vi "Statnett PMU Recorder Light.vi"(8 "error in (no error)":errorcluster) -> (0 "error out":errorcluster)   [LabVIEW 2013, in "PMU Recorder Light.lvlib"]
uses:
  PMU Recorder Light.lvlib
  <vilib>/Platform/TimedLoop/XDataNode/timing_clust.ctl
  <vilib>/Platform/TimedLoop/XDataNode/nitl_modes.ctl
  <vilib>/Platform/TimedLoop/XDataNode/wakeup.ctl
  <vilib>/Utility/sysdir.llb/System Directory Type.ctl
  <vilib>/platform/TimedLoop/XDataNode/XDataNode.xnode
  Phasor Data Concentrator Class/Phasor Data Concentrator.lvclass
  <vilib>/Platform/TimedLoop/XDataNode/XDNodeRunTimeDep.lvlib
panel:
  out "Number of bad dt":u64
  out "Latest Time Stamp":timestamp format="%<%X  %x>T"
  in  "Channel Selector":bool
  out "Manual Control":bool
  out "PDC Initialized":bool
  out "Queue Active":bool
  out "Connected":bool
  out "Configuration File Read":bool
  out "PDC Connected":bool
  out "Shutdown":bool
  out "Autostart":bool
  out "Bad Data Removal":bool
  out "Buffer Active":bool
  out "Configuration File Timeout":bool
  out "Configuration File Received":bool
  out "Initializing...":bool
  out "Bad Data?":bool
  out "Complex Bad":dbl(knob) scale=0.0..50.0
  out "Writing To File Buffer?":bool
  out "Lost File Buffer Data?":bool
  out "Writer Activity":dbl(knob) scale=0.0..100.0
  out "Buffer Queued?":bool
  out "Reader Activity":dbl(knob) scale=0.0..100.0
  out "Data?":bool
  out "Bad dt?":bool
  in  "Raw Data Panel":bool
  out "Worker Status":bool
  out "Secretary Pulse":bool
  out "Quitting...":bool
  out "Status":string="off"
  out "Data Rate":sgl=nan format="%#_6f"
  out "Control":enum32{"Auto", "Manual"}(tab)
  in  "Config":bool
  in  "Restart":bool
  in  "Quit":bool
  in  "Shutdown Logging":bool
  in  "Pause":bool
  in  "Startup":bool
  in  "Abort Wait":bool
  in  "PDC Initialize":bool
  in  "DLL Start Readers":bool
  in  "DLL Shutdown":bool
  in  "DLL Read Config":bool
  in  "DLL Wait for config":bool
  in  "DLL Initialize":bool
  in  "Quit 2":bool
  in  "Restart 2":bool
  in  "Config 2":bool
  in  "dt min":dbl=nan
  in  "dt max":dbl=nan
  in  "PRL Configuration":T1={"Connection Settings"={"IP-address"="127.0.0.1", "Port"="5001", "ID Code"=1001}, "Autostart"=FALSE, "Bad Data Removal"=TRUE, "Access Buffer Active"=TRUE, "Wait for Config Total Time [ms]"=2000, "Seconds to Wait if Config Fails [s]"=10, "Live Data Buffer Size"=5, "Number of Live Buffers in Access Buffer"=0, "Data Rate History"=100, "Complex Data Points Allowed Equal"=10, "Analog Data Points Allowed Equal"=50, "Number of Connection Attempts"=0, "Access Queue Active"=FALSE, "Access Buffer Size [hh:mm]"=600.0, "Sampling rate [Hz]"=nan, "Manual Control"=FALSE, "dt Tolerance [microseconds]"=10.0, "Wait for Config Timeout [ms]"=20, "Max Time Stamp Age Before Reconnect [s]"=10.0, "Poll New Data Timeout [ms]"=5} {"Access Buffer Size [hh:mm]" format="%<%H:%M>t"}
  # "INPUT"
  # "OUTPUT"
  # "INTERMEDIATE"
  # "v1.2  2013-08-01"
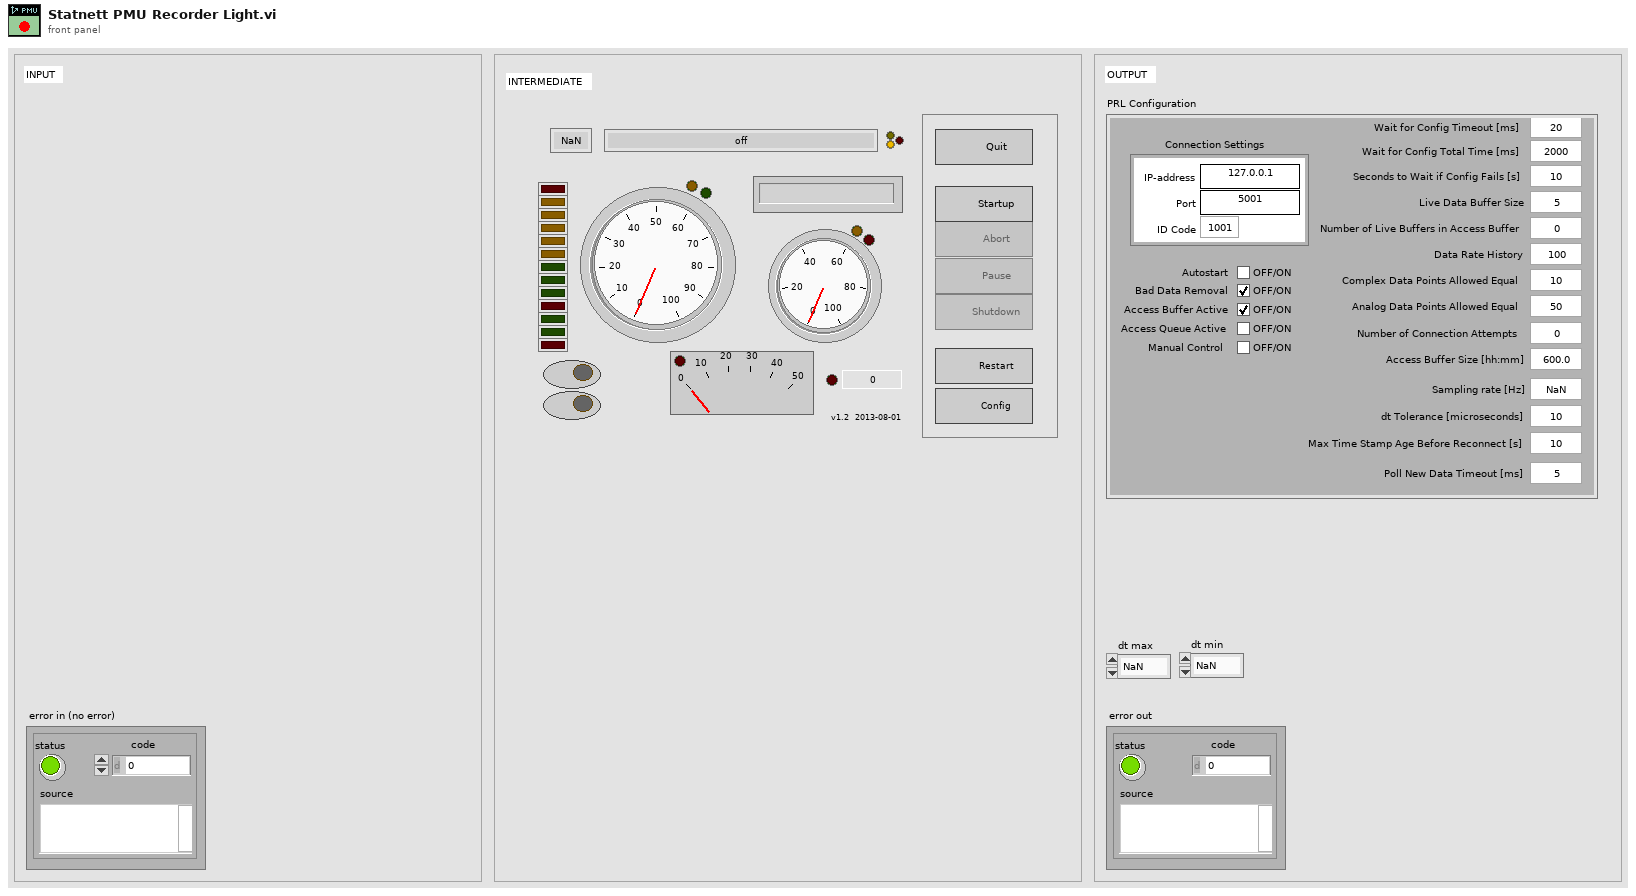
[diagram p1: front panel]
types:
  T1 = cluster{"Connection Settings":cluster{"IP-address":string, "Port":string, "ID Code":u32}, "Autostart":bool, "Bad Data Removal":bool, "Access Buffer Active":bool, "Wait for Config Total Time [ms]":i32, "Seconds to Wait if Config Fails [s]":i32, "Live Data Buffer Size":i32, "Number of Live Buffers in Access Buffer":i32, "Data Rate History":i32, "Complex Data Points Allowed Equal":i32, "Analog Data Points Allowed Equal":i32, "Number of Connection Attempts":i32, "Access Queue Active":bool, "Access Buffer Size [hh:mm]":dbl, "Sampling rate [Hz]":dbl, "Manual Control":bool, "dt Tolerance [microseconds]":dbl, "Wait for Config Timeout [ms]":i32, "Max Time Stamp Age Before Reconnect [s]":dbl, "Poll New Data Timeout [ms]":u16}
  T2 = typedef "XDNodeRunTimeDep.lvlib/timing_clust.ctl" = cluster{"Expected End [f-1]":u64, "Actual End [f-1]":u64, "Finished Late? [f-1]":bool, "Expected End [i-1]":u64, "Actual End [i-1]":u64, "Finished Late? [i-1]":bool, "Expected Start [i]":u64, "Actual Start [i]":u64, "Expected Start [f]":u64, "Actual Start [f]":u64, "Source Name":string, "Structure Name":string, "Period":i64, "Deadline":i64, "Offset":i64, "Start":i64, "Priority":i32, "Timeout":i32, "Mode":T3, "Wakeup Reason":T4, "Error":errorcluster, "Source Type":string, "Secondary Source Type":string, "Global End Time":u64, "Global Start Time":u64, "Frame Duration":u64, "Iteration Duration":u64, "Assigned CPU":i32, "I/O Scan Engine Mode":u32}
  T3 = typedef "XDNodeRunTimeDep.lvlib/nitl_modes.ctl" = enum32{"No Change", "Process missed periods, maintain original phase", "Discard missed periods, maintain original phase", "Process missed periods, ignore original phase", "Discard missed periods, ignore original phase"}
  T4 = typedef "XDNodeRunTimeDep.lvlib/wakeup.ctl" = enum32{"Normal", "Aborted", "Asynchronous wakeup", "Timing source error", "Timed loop error", "Timeout"}
  T5 = enum8{"Enabled", "Disabled", "Disabled and Grayed Out"}
  T6 = typedef "System Directory Type.ctl" = i32
  T7 = cluster{"IP-address":string, "Port":string, "ID Code":u32}
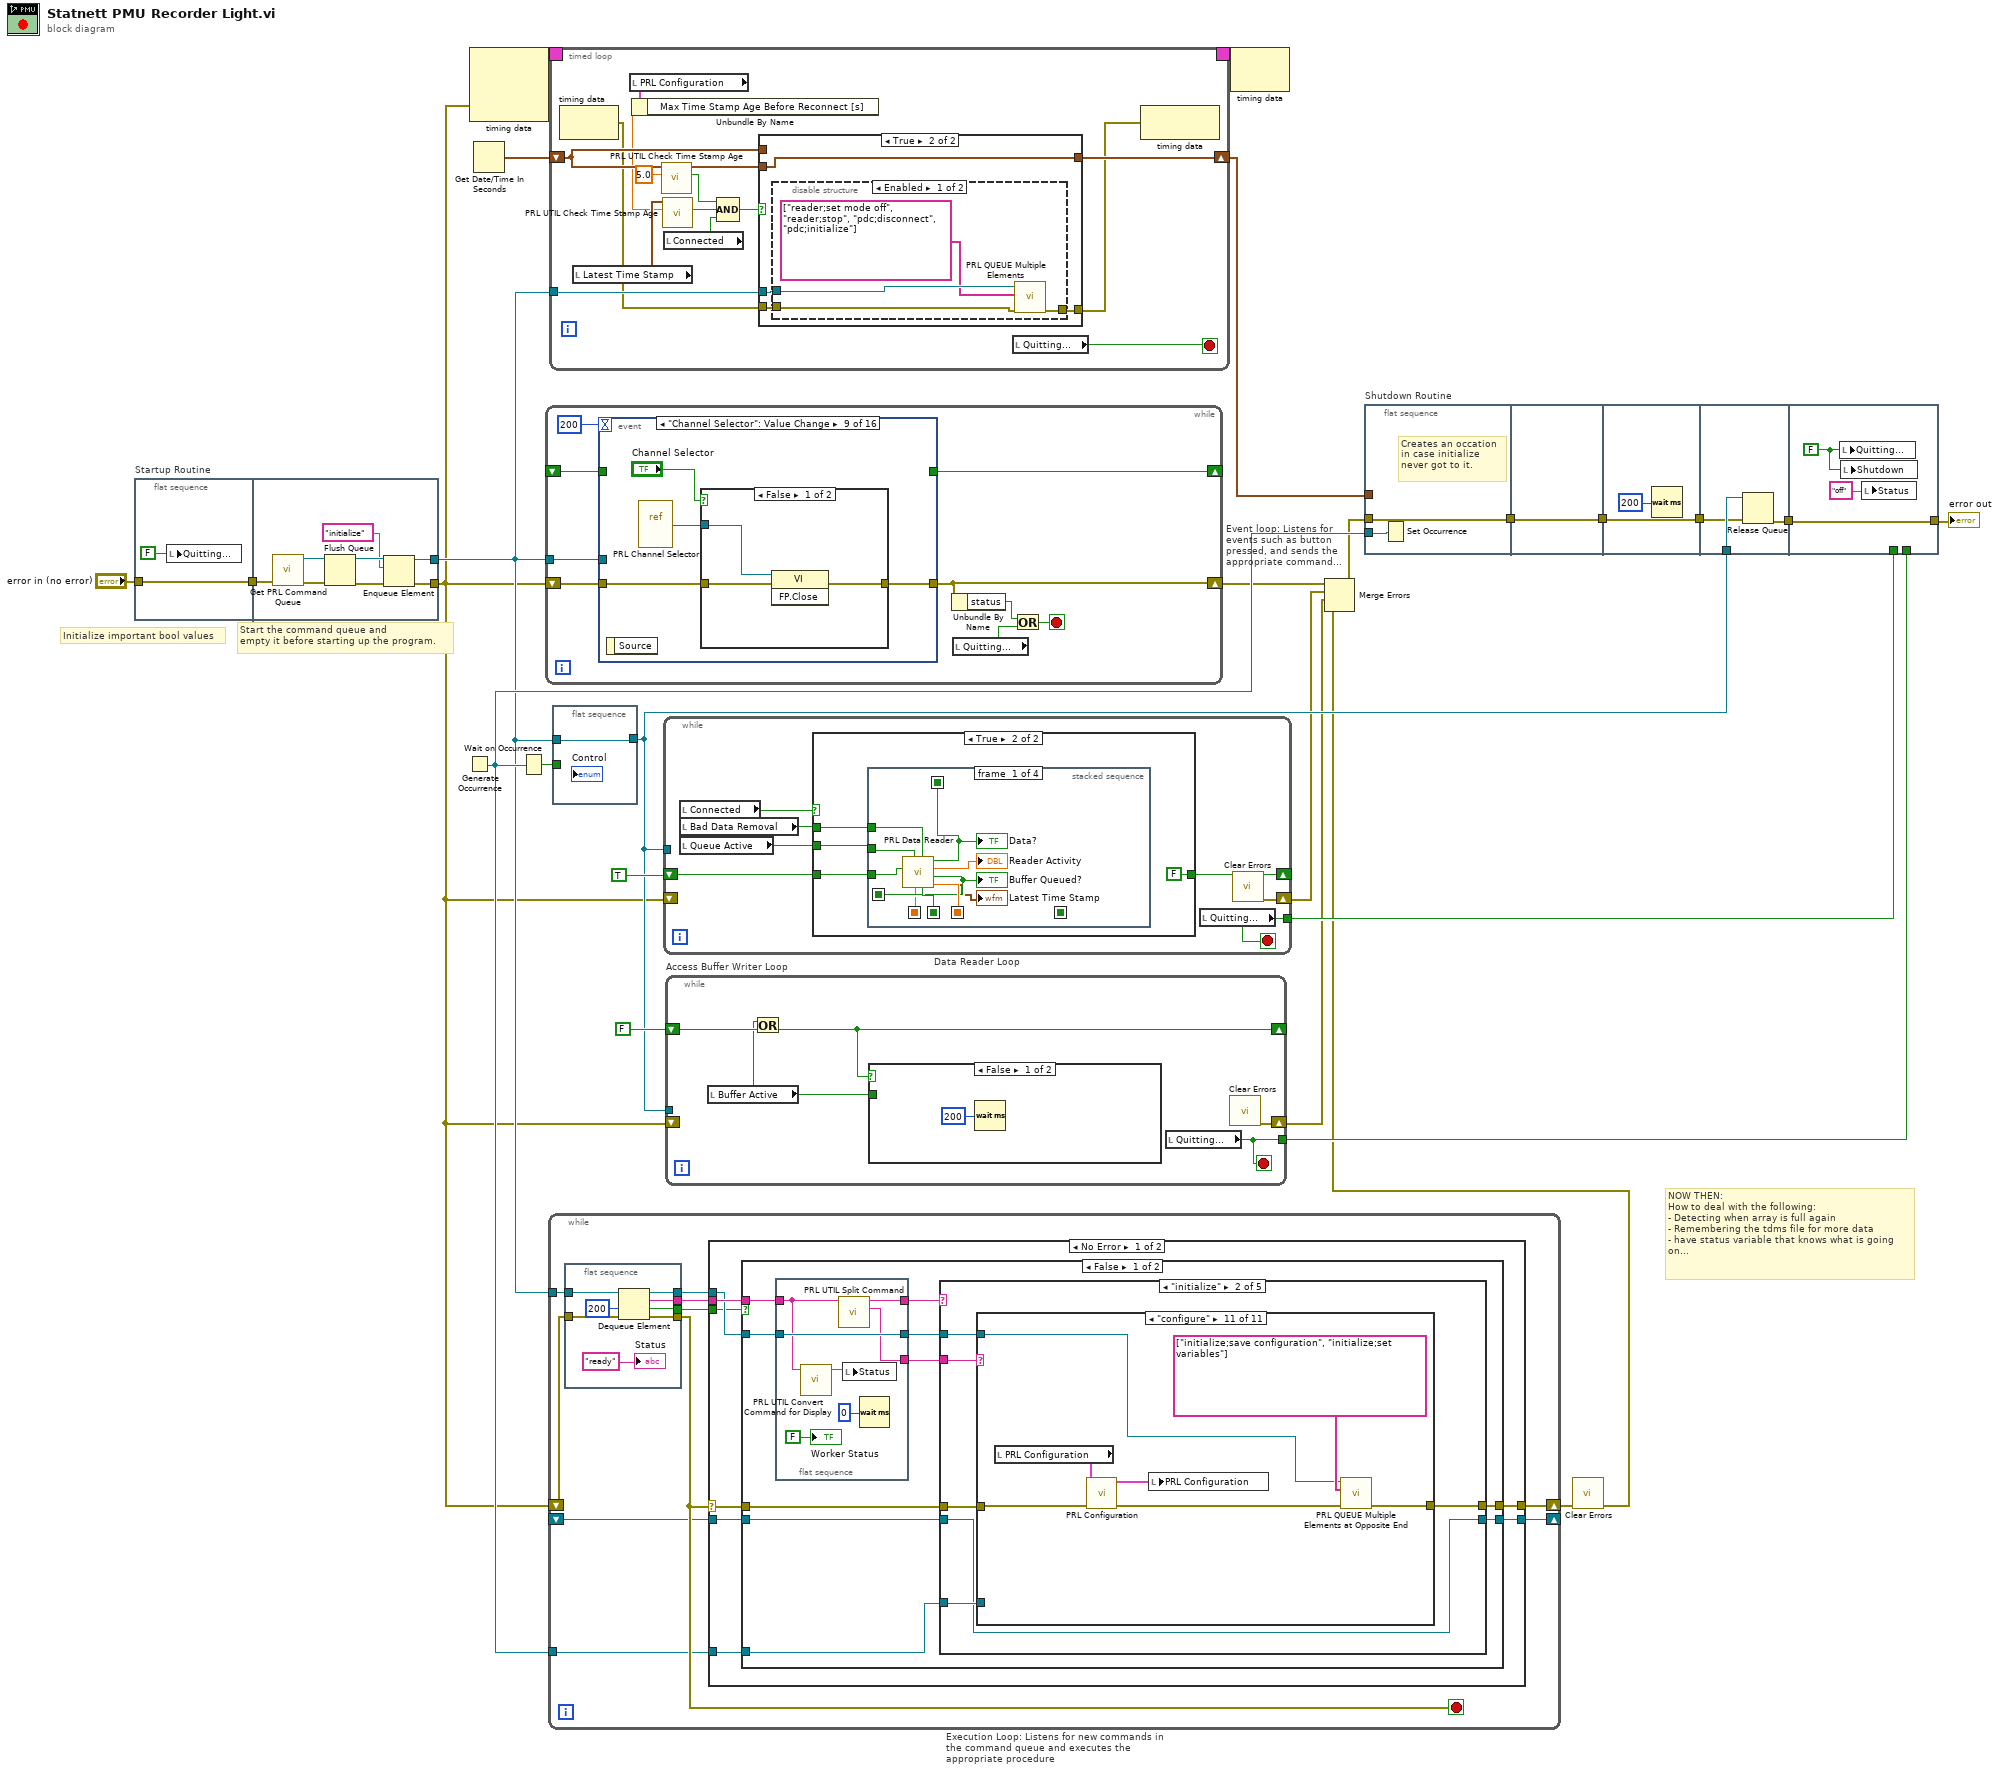
[diagram p0: block diagram]
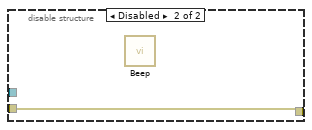
[diagram p3: hidden frame]
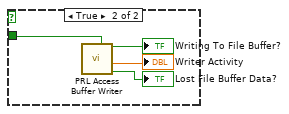
[diagram p4: hidden frame]
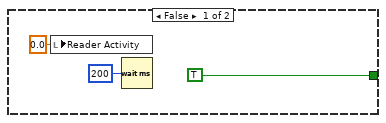
[diagram p5: hidden frame]
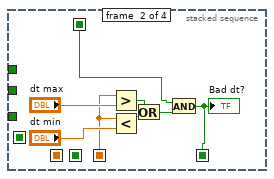
[diagram p6: hidden frame]
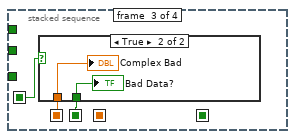
[diagram p7: hidden frame]
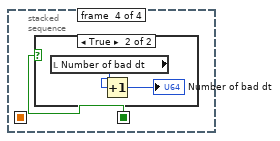
[diagram p9: hidden frame]
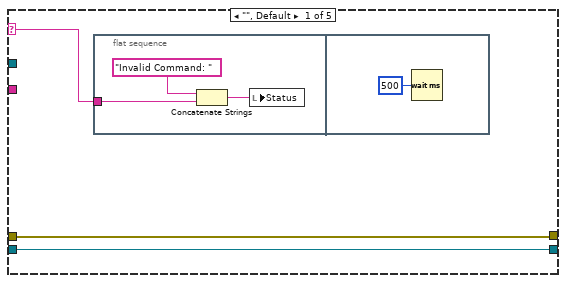
[diagram p11: hidden frame]
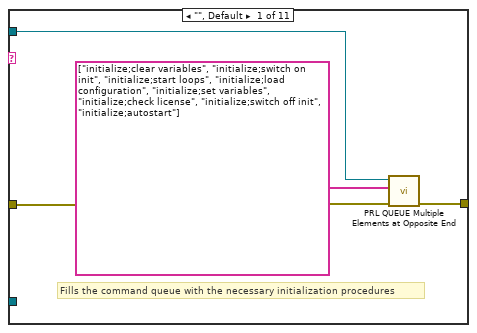
[diagram p12: hidden frame]
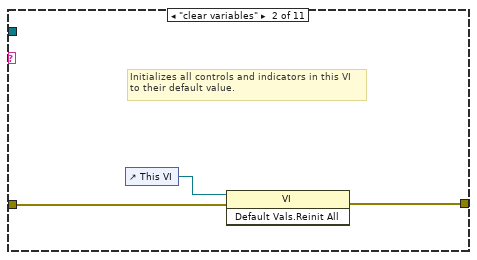
[diagram p13: hidden frame]
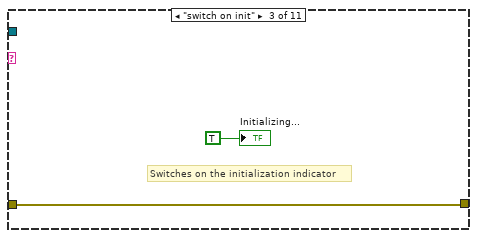
[diagram p14: hidden frame]
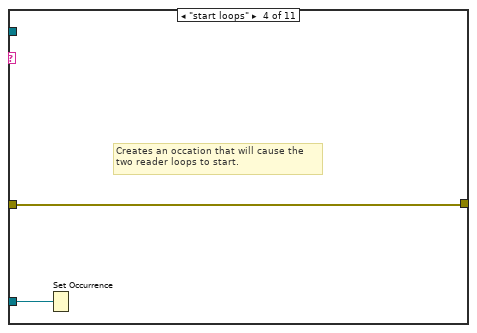
[diagram p15: hidden frame]
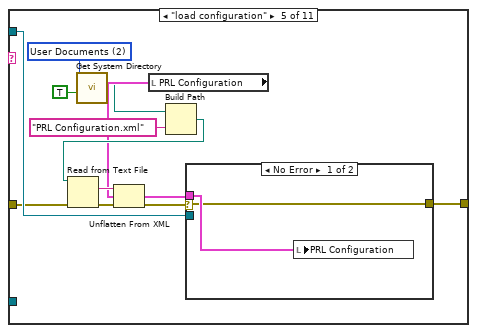
[diagram p16: hidden frame]
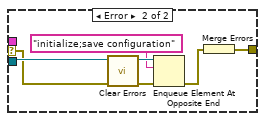
[diagram p17: hidden frame]
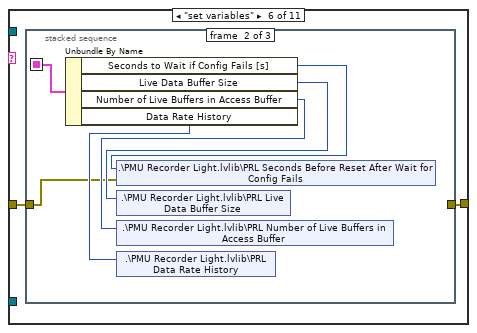
[diagram p18: hidden frame]
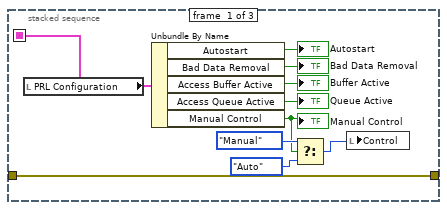
[diagram p19: hidden frame]
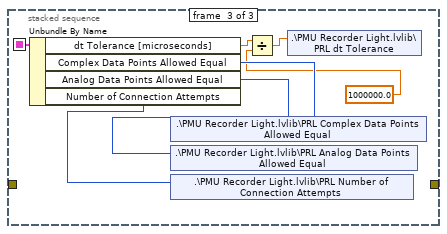
[diagram p20: hidden frame]
diagram:
  # "Initialize important bool values"
  # "Start the command queue and \nempty it before starting up the program."
  # "NOW THEN:\nHow to deal with the following:\n- Detecting when array is full again\n- Remembering the tdms file for more data\n- have status variable that knows what is going\non..."
  n1 = flat-sequence "Startup Routine" {
    tunnel: [w27] -> w14
    tunnel: "error in (no error)" -> [w27]
    tunnel: [w34] -> w10
    tunnel: [w32] -> w17
    tunnel: w14 -> [w29]
    frame #0 {
      n2 = local write "Quitting..."(FALSE ("Exit?")) -> ()
    }
    frame #1 {
      n3 = call "Get PRL Command Queue.vi"("error in (no error)"=w29) -> ("error out"=w30:errorcluster, "PRL Command Queue"=w31:refnum<queue>)  [unwired: 9 in]
      n4 = Flush Queue(queue=w31, error in (no error)=w30) -> (queue out=w35:refnum<queue>, error out=w36:errorcluster)  [unwired: 1 out]
      n5 = Enqueue Element(queue=w35, element="initialize", error in (no error)=w36) -> (queue out=w32:refnum<queue>, error out=w34:errorcluster)  [unwired: 2 out]
    }
  }
  n6 = Generate Occurrence() -> (w23:refnum<k4>)
  n7 = node-c288(w10) -> (w19:T2)  [unwired: 2 in]
  n8 = Get Date/Time In Seconds() -> (seconds since 1Jan1904=w16:timestamp)
  n9 = Wait on Occurrence(2:w23) -> (0:w24:bool)  [unwired: 2 in]
  n10 = while "Event loop: Listens for events such as button pressed, and sends the appropriate commands to the\ncommand queue" {
    shift-right: [w40] -> w9
    shift-left: w10 -> [w41]
    tunnel: w17 -> [w42]
    shift-right: [w37] -> _
    shift-left: _ -> [w38]
    stop <- w44 stop-if-true
    n11 = event shown="[8] \"Channel Selector\": Value Change" {
      selector: _ -> [_ _ _ _ _ _ _ _ _ _ _ _ _ _ _ _]
      dyn-events: _ -> [_ _ _ _ _ _ _ _ _ _ _ _ _ _ _ _]
      timeout: 200 -> [_ _ _ _ _ _ _ _ _ _ _ _ _ _ _ _]
      tunnel: w42 -> [_ w53 w57 w61 w65 w69 w76 _ _ w102 w106 w110 w114 w118 w122 w126]
      tunnel: [w48 w51 w55 w58 w63 w66 w74 w77 w88 w100 w103 w107 w112 w115 w119 w124] -> w40
      tunnel: w41 -> [w48 w52 w56 w59 w64 w67 w75 w78 w89 w101 w104 w108 w113 w116 w120 w125]
      tunnel: w38 -> [w47 _ _ _ _ _ _ _ _ _ _ _ _ _ _ _]
      tunnel: [w46 _ _ _ _ _ _ _ _ _ _ _ _ _ _ _] -> w37
      event Timeout {
        n12 = event-data() -> ()  [unwired: 3 out]
        n13 = Not(x=w47) -> (.not. x?=w46:bool)
        "Secretary Pulse" <- w47
      }
      event "Quit", "Quit 2": Value Change {
        n14 = event-data() -> ()  [unwired: 2 out]
        n15 = Enqueue Element(queue=w53, element="shutdown", error in (no error)=w52) -> (error out=w51:errorcluster)  [unwired: 3 out]
        "Shutdown" <- TRUE ("Shutdown")
      }
      event "Restart", "Restart 2": Value Change {
        n16 = event-data() -> ()  [unwired: 2 out]
        n17 = Enqueue Element(queue=w57, element="initialize", error in (no error)=w56) -> (error out=w55:errorcluster)  [unwired: 3 out]
      }
      event "Startup": Value Change {
        n18 = event-data() -> ()  [unwired: 2 out]
        n19 = call "PRL QUEUE Multiple Elements.vi"("error in"=w59, "Elements to Add"=string[] ["pdc;initialize"], "queue"=w61) -> ("error out"=w58:errorcluster)  [unwired: 7 in, 1 out]
      }
      event "PDC Initialize": Value Change {
        n20 = event-data() -> ()  [unwired: 2 out]
        n21 = Enqueue Element(queue=w65, element="pdc;init", error in (no error)=w64) -> (error out=w63:errorcluster)  [unwired: 3 out]
      }
      event "Shutdown Logging": Value Change {
        n22 = event-data() -> ()  [unwired: 2 out]
        n23 = call "PRL QUEUE Multiple Elements.vi"("error in"=w67, "Elements to Add"=string[] ["reader;set mode off", "reader;stop", "pdc;disconnect"], "queue"=w69) -> ("error out"=w66:errorcluster)  [unwired: 7 in, 1 out]
      }
      event "Pause": Value Change {
        n24 = event-data() -> ()  [unwired: 2 out]
        n25 = Select(t=string[] ["reader;set mode paused", "reader;stop"] ("Elements to Add"), s="Pause", f=string[] ["reader;start", "reader;set mode logging"] ("Elements to Add")) -> (s? t:f=w71:string[])
        n26 = call "PRL QUEUE Multiple Elements.vi"("error in"=w75, "Elements to Add"=w71, "queue"=w76) -> ("error out"=w74:errorcluster)  [unwired: 7 in, 1 out]
      }
      event "Raw Data Panel": Value Change {
        n27 = event-data() -> ()  [unwired: 2 out]
        n28 = vi-ref "PRL Raw Data Viewer.vi"() -> (w80:refnum<vi>)
        n29 = case shown="True" "Raw Data Panel" {
          tunnel: w80 -> [w83 w87]
          tunnel: [w82 w85] -> w77
          tunnel: w78 -> [w81 w84]
          frame False {
            n30 = invoke class="VI" method="FP.Close"(reference=w83, error in=w81) -> (error out=w82:errorcluster)  [unwired: 1 in, 2 out]
          }
          frame True {
            n31 = invoke class="VI" method="FP.Open"(reference=w87, error in=w84, "Activate"=TRUE ("Activate?")) -> (error out=w85:errorcluster)  [unwired: 2 in, 4 out]
          }
        }
      }
      event "Channel Selector": Value Change {
        n32 = event-data() -> ()  [unwired: 2 out]
        n33 = vi-ref "PRL Channel Selector.vi"() -> (w91:refnum<vi>)
        n34 = case shown="False" "Channel Selector" {
          tunnel: w91 -> [w94 w98]
          tunnel: [w93 w96] -> w88
          tunnel: w89 -> [w92 w95]
          frame False {
            n35 = invoke class="VI" method="FP.Close"(reference=w94, error in=w92) -> (error out=w93:errorcluster)  [unwired: 1 in, 2 out]
          }
          frame True {
            n36 = invoke class="VI" method="FP.Open"(reference=w98, error in=w95, "Activate"=TRUE ("Activate?")) -> (error out=w96:errorcluster)  [unwired: 2 in, 4 out]
          }
        }
      }
      event "Config", "Config 2": Value Change {
        n37 = event-data() -> ()  [unwired: 2 out]
        n38 = Enqueue Element(queue=w102, element="initialize;configure", error in (no error)=w101) -> (error out=w100:errorcluster)  [unwired: 3 out]
      }
      event "DLL Initialize": Value Change {
        n39 = event-data() -> ()  [unwired: 2 out]
        n40 = Enqueue Element(queue=w106, element="pdc;dll initialize", error in (no error)=w104) -> (error out=w103:errorcluster)  [unwired: 3 out]
      }
      event "DLL Wait for config": Value Change {
        n41 = event-data() -> ()  [unwired: 2 out]
        n42 = Enqueue Element(queue=w110, element="pdc;dll wait for config", error in (no error)=w108) -> (error out=w107:errorcluster)  [unwired: 3 out]
      }
      event "DLL Start Readers": Value Change {
        n43 = event-data() -> ()  [unwired: 2 out]
        n44 = Enqueue Element(queue=w114, element="pdc;start data readers", error in (no error)=w113) -> (error out=w112:errorcluster)  [unwired: 3 out]
      }
      event "DLL Read Config": Value Change {
        n45 = event-data() -> ()  [unwired: 2 out]
        n46 = Enqueue Element(queue=w118, element="pdc;dll read config", error in (no error)=w116) -> (error out=w115:errorcluster)  [unwired: 3 out]
      }
      event "DLL Shutdown": Value Change {
        n47 = event-data() -> ()  [unwired: 2 out]
        n48 = Enqueue Element(queue=w122, element="pdc;disconnect", error in (no error)=w120) -> (error out=w119:errorcluster)  [unwired: 3 out]
      }
      event "Abort Wait": Value Change {
        n49 = event-data() -> ()  [unwired: 2 out]
        n50 = Enqueue Element(queue=w126, element="reader;set mode startup", error in (no error)=w125) -> (error out=w124:errorcluster)  [unwired: 3 out]
      }
    }
    n51 = Unbundle By Name(w40) -> ("status"=w45:bool)
    n52 = local read "Quitting..."() -> (w43:bool)
    n53 = Or(x=w45, y=w43) -> (x .or. y?=w44:bool)
  }
  n54 = while "Execution Loop: Listens for new commands in the command queue and executes the appropriate procedure" {
    tunnel: w17 -> [w136]
    tunnel: w23 -> [w131]
    shift-right: [w129] -> _
    shift-left: _ -> [w130]
    shift-right: [w127] -> w2
    shift-left: w10 -> [w128]
    stop <- w133 stop-if-true
    n55 = flat-sequence {
      tunnel: w136 -> [w144]
      tunnel: [w143] -> w135
      tunnel: [w142] -> w134
      tunnel: [w141] -> w133
      tunnel: [w138] -> w132
      tunnel: w128 -> [w137]
      frame #0 {
        n56 = Dequeue Element(queue=w144, timeout in ms (-1)=200, error in (no error)=w137) -> (queue out=w143:refnum<queue>, element=w142:string, timed out?=w138:bool, error out=w141:errorcluster)
        "Status" <- "ready" ("Status")
      }
    }
    n57 = case shown="No Error" w133 {
      selector: w133 -> [w146 w502]
      tunnel: w135 -> [w151 _]
      tunnel: w134 -> [w152 _]
      tunnel: w132 -> [w150 _]
      tunnel: w131 -> [w149 _]
      tunnel: w130 -> [w148 w503]
      tunnel: [w147 w503] -> w129
      tunnel: [w145 w502] -> w127
      frame No Error {
        n58 = case shown="False" w150 {
          tunnel: w152 -> [w162 _]
          tunnel: w151 -> [w161 _]
          tunnel: w149 -> [w157 _]
          tunnel: w148 -> [w156 w499]
          tunnel: [w155 w499] -> w147
          tunnel: w146 -> [w154 w498]
          tunnel: [w153 w498] -> w145
          frame False {
            n59 = flat-sequence {
              tunnel: [w495] -> w160
              tunnel: w162 -> [w493]
              tunnel: w161 -> [w497]
              tunnel: [w497] -> w159
              tunnel: [w494] -> w158
              frame #0 {
                n60 = call "PRL UTIL Convert Command for Display.vi"("Command In"=w493) -> ("Command Out"=w492:string)  [unwired: 10 in]
                n61 = call "PRL UTIL Split Command.vi"("Command"=w493) -> ("Parameters"=w494:string, "Command Out"=w495:string)  [unwired: 9 in]
                n62 = local write "Status"(w492) -> ()
                n63 = Wait (ms)(milliseconds to wait=u32 0) -> ()  [unwired: 1 out]
                "Worker Status" <- FALSE ("System Ready")
              }
            }
            n64 = case shown="\"initialize\"" w160 {
              selector: w160 -> [w165 _ _ _ _]
              tunnel: w159 -> [_ w175 w269 w421 w482]
              tunnel: w158 -> [_ w174 w270 w422 w481]
              tunnel: w157 -> [_ w173 _ _ _]
              tunnel: w156 -> [w164 w172 w268 w420 w480]
              tunnel: [w164 w172 w267 w420 w480] -> w155
              tunnel: w154 -> [w163 w171 w266 w419 w479]
              tunnel: [w163 w170 w265 w418 w478] -> w153
              frame "", Default {
                n65 = flat-sequence {
                  tunnel: w165 -> [w167]
                  frame #0 {
                    n66 = Concatenate Strings("Invalid Command: " ("Status"), w167) -> (w166:string)
                    n67 = local write "Status"(w166) -> ()
                  }
                  frame #1 {
                    n68 = Wait (ms)(milliseconds to wait=u32 500) -> ()  [unwired: 1 out]
                  }
                }
              }
              frame "initialize" {
                n69 = case shown="\"configure\"" w174 {
                  tunnel: w175 -> [w179 _ _ _ w193 _ _ _ _ w254 w258]
                  tunnel: w173 -> [_ _ _ w186 _ _ _ _ _ _ _]
                  tunnel: w171 -> [w177 w181 w183 w185 w188 w209 w233 w241 w249 w252 w260]
                  tunnel: [w176 w180 w183 w185 w187 w208 w234 w240 w249 w251 w261] -> w170
                  frame "", Default {
                    # "Fills the command queue with the necessary initialization procedures"
                    n70 = call "PRL QUEUE Multiple Elements at Opposite End.vi"("error in"=w177, "Elements to Add"=string[] ["initialize;clear variables", "initialize;switch on init", "initialize;start loops", "initialize;load configuration", "initialize;set variables", "initialize;check license", "initialize;switch off init", "initialize;autostart"], "queue"=w179) -> ("error out"=w176:errorcluster)  [unwired: 7 in, 1 out]
                  }
                  frame "clear variables" {
                    # "Initializes all controls and indicators in this VI\nto their default value."
                    n71 = control-ref of="This VI"() -> (w182:refnum<vi>)
                    n72 = invoke class="VI" method="Default Vals.Reinit All"(reference=w182, error in=w181) -> (error out=w180:errorcluster)  [unwired: 1 in, 2 out]
                  }
                  frame "switch on init" {
                    # "Switches on the initialization indicator"
                    "Initializing..." <- TRUE ("Initializing...")
                  }
                  frame "start loops" {
                    # "Creates an occation that will cause the \ntwo reader loops to start."
                    n73 = Set Occurrence(w186) -> ()
                  }
                  frame "load configuration" {
                    w191 = T6 2 items=["User Home"=0, "User Desktop"=1, "User Documents"=2, "User Application Data"=3, "User Preferences"=4, "User Temporary"=5, "Public Documents"=6, "Public Application Data"=7, "Public Preferences"=8, "Public Cache"=13, "System Core Libraries"=9, "System Installed Libraries"=10, "Application Files"=11, "Boot Volume Root"=12] ("system directory type")
                    n74 = call <vilib>:"Get System Directory.vi"("create directory if not found? (F)"=TRUE, "system directory type"=w191) -> ("system directory"=w189:path)  [unwired: 9 in]
                    n75 = local read "PRL Configuration"() -> (w195:T1)
                    n76 = Build Path(base path=w189, name or relative path="PRL Configuration.xml") -> (appended path=w196:path)
                    n77 = Read from Text File(file (use dialog)=w196, error in=w188) -> (text=w199:string, error out=w198:errorcluster)  [unwired: 2 in, 2 out]
                    n78 = Unflatten From XML(xml string=w199, type=w195, error in (no error)=w198) -> (value=w192:T1, error out=w194:errorcluster)
                    n79 = case shown="No Error" w194 {
                      selector: w194 -> [w200 w204]
                      tunnel: w193 -> [_ w207]
                      tunnel: w192 -> [w201 _]
                      tunnel: [w200 w202] -> w187
                      frame No Error {
                        n80 = local write "PRL Configuration"(w201) -> ()
                      }
                      frame Error {
                        n81 = call <vilib>:"Clear Errors.vi"("error in (no error)"=w204) -> ("error out"=w205:errorcluster)  [unwired: 6 in]
                        n82 = Enqueue Element At Opposite End(queue=w207, element="initialize;save configuration", error in (no error)=w205) -> (error out=w203:errorcluster)  [unwired: 1 in, 2 out]
                        n83 = Merge Errors(w203) -> (w202:errorcluster)
                      }
                    }
                  }
                  frame "set variables" {
                    n84 = stacked-sequence {
                      seq-local: [w216 _ _] -> [_ w225 w232]
                      tunnel: w209 -> [w210 w220 _]
                      tunnel: [w210 _ _] -> w208
                      frame #0 {
                        n85 = local read "PRL Configuration"() -> (w216:T1)
                        n86 = Unbundle By Name(w216) -> ("Autostart"=→"Autostart":bool, "Bad Data Removal"=→"Bad Data Removal":bool, "Access Buffer Active"=→"Buffer Active":bool, "Access Queue Active"=→"Queue Active":bool, "Manual Control"=w211:bool)
                        "Manual Control" <- w211
                        n87 = Select(t=enum32{"Auto", "Manual"}."Manual" ("Control"), s=w211, f=enum32{"Auto", "Manual"}."Auto" ("Control")) -> (s? t:f=w214:enum32{"Auto", "Manual"})
                        n88 = local write "Control"(w214) -> ()
                      }
                      frame #1 {
                        n89 = Unbundle By Name(w225) -> ("Seconds to Wait if Config Fails [s]"=w224:i32, "Live Data Buffer Size"=w222:i32, "Number of Live Buffers in Access Buffer"=w221:i32, "Data Rate History"=w223:i32)
                        n90 = shared-variable ".\\PMU Recorder Light.lvlib\\PRL Seconds Before Reset After Wait for Config Fails"(w224, error in=w220) -> ()  [unwired: 1 out]
                        n91 = shared-variable ".\\PMU Recorder Light.lvlib\\PRL Live Data Buffer Size"(w222) -> ()  [unwired: 1 in, 1 out]
                        n92 = shared-variable ".\\PMU Recorder Light.lvlib\\PRL Number of Live Buffers in Access Buffer"(w221) -> ()  [unwired: 1 in, 1 out]
                        n93 = shared-variable ".\\PMU Recorder Light.lvlib\\PRL Data Rate History"(w223) -> ()  [unwired: 1 in, 1 out]
                      }
                      frame #2 {
                        n94 = Unbundle By Name(w232) -> ("dt Tolerance [microseconds]"=w228:dbl, "Complex Data Points Allowed Equal"=w230:i32, "Analog Data Points Allowed Equal"=w231:i32, "Number of Connection Attempts"=w229:i32)
                        n95 = shared-variable ".\\PMU Recorder Light.lvlib\\PRL Complex Data Points Allowed Equal"(w230) -> ()  [unwired: 1 in, 1 out]
                        n96 = shared-variable ".\\PMU Recorder Light.lvlib\\PRL Analog Data Points Allowed Equal"(w231) -> ()  [unwired: 1 in, 1 out]
                        n97 = shared-variable ".\\PMU Recorder Light.lvlib\\PRL Number of Connection Attempts"(w229) -> ()  [unwired: 1 in, 1 out]
                        n98 = Divide(x=w228, y=1000000.0) -> (x/y=w226:dbl)
                        n99 = shared-variable ".\\PMU Recorder Light.lvlib\\PRL dt Tolerance"(w226) -> ()  [unwired: 1 in, 1 out]
                      }
                    }
                  }
                  frame "check license" {
                    n100 = disable-structure shown="Enabled" {
                      disable-tunnel: [_ w239] -> w234
                      disable-tunnel: w233 -> [_ w239]
                      frame Disabled {
                        n101 = Get Date/Time In Seconds() -> (seconds since 1Jan1904=w237:timestamp)
                        n102 = Greater Or Equal?(x=w237, y=timestamp(3471375600 s since 1904-01-01)) -> (x >= y?=w235:bool)
                        n103 = case shown="True" w235 {
                          frame False {
                          }
                          frame True {
                            n104 = One Button Dialog(message="This version of the software \nis not licensed for use after \nJanuary 1st 2014.\n\nPlease contact Statnett R&D\nfor an upgrade.") -> ()  [unwired: 1 in, 1 out]
                          }
                        }
                      }
                      frame Enabled {
                        # "No License Check"
                      }
                    }
                  }
                  frame "save configuration" {
                    w244 = T6 2 items=["User Home"=0, "User Desktop"=1, "User Documents"=2, "User Application Data"=3, "User Preferences"=4, "User Temporary"=5, "Public Documents"=6, "Public Application Data"=7, "Public Preferences"=8, "Public Cache"=13, "System Core Libraries"=9, "System Installed Libraries"=10, "Application Files"=11, "Boot Volume Root"=12] ("system directory type")
                    n105 = call <vilib>:"Get System Directory.vi"("create directory if not found? (F)"=TRUE, "system directory type"=w244) -> ("system directory"=w242:path)  [unwired: 9 in]
                    n106 = Build Path(base path=w242, name or relative path="PRL Configuration.xml") -> (appended path=w246:path)
                    n107 = Flatten To XML(anything="PRL Configuration") -> (xml string=w247:string)
                    n108 = Write to Text File(file (use dialog)=w246, text=w247, error in=w241) -> (error out=w240:errorcluster)  [unwired: 1 in, 2 out]
                  }
                  frame "switch off init" {
                    n109 = local write "Initializing..."(FALSE ("Init")) -> ()
                  }
                  frame "autostart" {
                    n110 = local read "Autostart"() -> (w255:bool)
                    n111 = Select(t=string[] ["pdc;initialize"] ("Elements to Add"), s=w255, f=string[] ["reader;set mode off"] ("Elements to Add")) -> (s? t:f=w253:string[])
                    n112 = call "PRL QUEUE Multiple Elements.vi"("error in"=w252, "Elements to Add"=w253, "queue"=w254) -> ("error out"=w251:errorcluster)  [unwired: 7 in, 1 out]
                  }
                  frame "configure" {
                    n113 = local read "PRL Configuration"() -> (w264:T1)
                    n114 = call "PRL Configuration.vi"("Error In"=w260, "Configuration In"=w264) -> ("Error Out"=w259:errorcluster, "Configuration Out"=w263:T1)  [unwired: 8 in]
                    n115 = local write "PRL Configuration"(w263) -> ()
                    n116 = call "PRL QUEUE Multiple Elements at Opposite End.vi"("error in"=w259, "Elements to Add"=string[] ["initialize;save configuration", "initialize;set variables"], "queue"=w258) -> ("error out"=w261:errorcluster)  [unwired: 7 in, 1 out]
                  }
                }
              }
              frame "pdc" {
                n117 = case shown="\"initialize\", Default" w270 {
                  tunnel: w269 -> [w275 _ w299 w319 w335 w357 w387 _ _ _]
                  tunnel: w268 -> [w273 _ w297 w317 w343 w364 w388 w392 w396 w402]
                  tunnel: [w273 w282 w289 w317 w337 w358 w384 w391 w395 w401] -> w267
                  tunnel: w266 -> [w272 w277 w291 w312 w334 w354 w378 w390 w394 w400]
                  tunnel: [w271 w276 w287 w311 w332 w352 w376 w389 w393 w399] -> w265
                  frame "initialize", Default {
                    n118 = call "PRL QUEUE Multiple Elements at Opposite End.vi"("error in"=w272, "Elements to Add"=string[] ["reader;set mode startup", "pdc;init object", "pdc;connect"], "queue"=w275) -> ("error out"=w271:errorcluster)  [unwired: 7 in, 1 out]
                  }
                  frame "init object" {
                    n119 = local read "PRL Configuration"() -> (w285:T1)
                    n120 = Unbundle By Name(w285) -> ("Connection Settings"=w284:T7, "Wait for Config Timeout [ms]"=w283:i32, "Wait for Config Total Time [ms]"=w279:i32)
                    n121 = control-ref of="Abort Wait"() -> (w278:refnum<vi>)
                    n122 = control-ref of="Quitting..."() -> (w280:refnum<vi>)
                    n123 = local write "Complex Bad"(0.0 ("Complex Bad")) -> ()
                    n124 = call "New.vi"("Abort Wait Reference 2"=w278, "Abort Wait Reference"=w280, "error in (no error)"=w277, "Wait for Config Total Time [ms]"=w279, "Wait for Config Timeout [ms]"=w283, "Connection Settings"=w284) -> ("error out"=w276:errorcluster, "Phasor Data Concentrator out"=w282:refnum<class "Phasor Data Concentrator.lvclass">)  [unwired: 4 in]
                    "PDC Initialized" <- TRUE ("PDC Initialized")
                  }
                  frame "connect" {
                    n125 = call "DLL Connect.vi"("error in (no error)"=w291, "Phasor Data Concentrator in"=w297) -> ("error out"=w296:errorcluster, "Phasor Data Concentrator out"=w298:refnum<class "Phasor Data Concentrator.lvclass">)  [unwired: 8 in]
                    n126 = call "DLL Get Status.vi"("error in (no error)"=w296, "Phasor Data Concentrator in"=w298) -> ("error out"=w290:errorcluster, "Configuration File Received"=→"Configuration File Received":bool, "Timeout"=→"Configuration File Timeout":bool, "Phasor Data Concentrator out"=w288:refnum<class "Phasor Data Concentrator.lvclass">, "Configuration Read OK"=→"Configuration File Read":bool, "PDC Connected"=w293:bool, "Data Rate"=→"Data Rate":sgl)  [unwired: 3 in]
                    "PDC Connected" <- w293
                    n127 = case shown="False" w293 {
                      tunnel: w299 -> [w304 w310]
                      tunnel: w290 -> [w302 w307]
                      tunnel: [w303 w308] -> w289
                      tunnel: w288 -> [w303 w308]
                      tunnel: [w301 w306] -> w287
                      frame False {
                        # "PDC Not Connected, so retrying"
                        n128 = call "PRL QUEUE Multiple Elements.vi"("error in"=w302, "Elements to Add"=string[] ["reader;set mode startup", "pdc;disconnect", "pdc;wait before reconnect"], "queue"=w304) -> ("error out"=w301:errorcluster)  [unwired: 7 in, 1 out]
                      }
                      frame True {
                        # "PDC Connected OK, so\nwaiting for config"
                        n129 = Enqueue Element(queue=w310, element="pdc;wait for config", error in (no error)=w307) -> (error out=w306:errorcluster)  [unwired: 3 out]
                      }
                    }
                  }
                  frame "wait before reconnect" {
                    n130 = shared-variable ".\\PMU Recorder Light.lvlib\\PRL Seconds Before Reset After Wait for Config Fails"() -> (w318:i32)  [unwired: 1 in, 1 out]
                    n131 = Tick Count (ms)() -> (millisecond timer value=w321:u32)
                    n132 = Multiply(x=w318, y=1000) -> (x*y=w320:i32)
                    n133 = while {
                      tunnel: w321 -> [w329]
                      tunnel: w320 -> [w327]
                      tunnel: [w325] -> w316
                      stop <- w326 stop-if-true
                      n134 = Tick Count (ms)() -> (millisecond timer value=w330:u32)
                      n135 = local read "Shutdown"() -> (w324:bool)
                      n136 = local read "Abort Wait"() -> (w323:bool)
                      n137 = Subtract(x=w330, y=w329) -> (x-y=w328:u32)
                      n138 = Greater?(x=w328, y=w327) -> (0:w325:bool)
                      n139 = Wait (ms)(milliseconds to wait=u32 20) -> ()  [unwired: 1 out]
                      n140 = Compound Arithmetic op=OR(w325, w324, w323) -> (w326:bool)
                    }
                    n141 = Select(t=string[] ["pdc;initialize", "reader;set mode logging"] ("Elements to Add"), s=w316, f=string[] ["reader;set mode off"] ("Elements to Add")) -> (s? t:f=w313:string[])
                    n142 = call "PRL QUEUE Multiple Elements.vi"("error in"=w312, "Elements to Add"=w313, "queue"=w319) -> ("error out"=w311:errorcluster)  [unwired: 7 in, 1 out]
                  }
                  frame "wait for config" {
                    n143 = call "DLL Wait for Config.vi"("error in (no error)"=w334, "Phasor Data Concentrator in"=w343) -> ("error out"=w338:errorcluster, "Phasor Data Concentrator out"=w339:refnum<class "Phasor Data Concentrator.lvclass">)  [unwired: 8 in]
                    n144 = call "DLL Get Status.vi"("error in (no error)"=w338, "Phasor Data Concentrator in"=w339) -> ("error out"=w333:errorcluster, "Configuration File Received"=w336:bool, "Timeout"=w340:bool, "Phasor Data Concentrator out"=w337:refnum<class "Phasor Data Concentrator.lvclass">, "Configuration Read OK"=w341:bool, "PDC Connected"=w342:bool)  [unwired: 3 in, 1 out]
                    n145 = case shown="False" w336 {
                      tunnel: w335 -> [w346 w351]
                      tunnel: w333 -> [w345 w349]
                      tunnel: [w344 w348] -> w332
                      frame False {
                        # "Configuration not received, so retrying..."
                        n146 = call "PRL QUEUE Multiple Elements.vi"("error in"=w345, "Elements to Add"=string[] ["reader;set mode startup", "pdc;disconnect", "pdc;wait before reconnect"], "queue"=w346) -> ("error out"=w344:errorcluster)  [unwired: 7 in, 1 out]
                      }
                      frame True {
                        # "Configuration received OK,\nso reading config"
                        n147 = Enqueue Element(queue=w351, element="pdc;read config", error in (no error)=w349) -> (error out=w348:errorcluster)  [unwired: 3 out]
                      }
                    }
                    n148 = local write "PDC Connected"(w342) -> ()
                    n149 = local write "Configuration File Timeout"(w340) -> ()
                    n150 = local write "Configuration File Received"(w336) -> ()
                    n151 = local write "Configuration File Read"(w341) -> ()
                  }
                  frame "read config" {
                    n152 = call "DLL Read Config.vi"("error in (no error)"=w354, "Phasor Data Concentrator in"=w364) -> ("error out"=w359:errorcluster, "Phasor Data Concentrator out"=w360:refnum<class "Phasor Data Concentrator.lvclass">)  [unwired: 8 in]
                    n153 = call "DLL Get Status.vi"("error in (no error)"=w359, "Phasor Data Concentrator in"=w360) -> ("error out"=w353:errorcluster, "Configuration File Received"=w362:bool, "Timeout"=w361:bool, "Phasor Data Concentrator out"=w358:refnum<class "Phasor Data Concentrator.lvclass">, "Configuration Read OK"=w356:bool, "PDC Connected"=w363:bool, "Data Rate"=w355:sgl)  [unwired: 3 in]
                    n154 = case shown="False" w356 {
                      tunnel: w357 -> [w367 w375]
                      tunnel: w355 -> [_ w372]
                      tunnel: w353 -> [w366 w370]
                      tunnel: [w365 w369] -> w352
                      frame False {
                        # "Configuration not read, so retrying..."
                        n155 = call "PRL QUEUE Multiple Elements.vi"("error in"=w366, "Elements to Add"=string[] ["reader;set mode startup", "pdc;disconnect", "pdc;wait before reconnect"], "queue"=w367) -> ("error out"=w365:errorcluster)  [unwired: 7 in, 1 out]
                      }
                      frame True {
                        # "Configuration read OK,\nso initializing readers"
                        n156 = local read "PRL Configuration"() -> (w373:T1)
                        n157 = Bundle By Name(cluster=w373, "Sampling rate [Hz]"=w372) -> (w371:T1)
                        n158 = local write "PRL Configuration"(w371) -> ()
                        n159 = Enqueue Element(queue=w375, element="pdc;initialize data readers", error in (no error)=w370) -> (error out=w369:errorcluster)  [unwired: 3 out]
                      }
                    }
                    n160 = local write "Data Rate"(w355) -> ()
                    n161 = local write "PDC Connected"(w363) -> ()
                    n162 = local write "Configuration File Timeout"(w361) -> ()
                    n163 = local write "Configuration File Received"(w362) -> ()
                    n164 = local write "Configuration File Read"(w356) -> ()
                  }
                  frame "initialize data readers" {
                    # "Initialize\n- Access Buffer Writer\n- DLL readers with number of channels\n- Data Reader with number of channels\n- Data Selector with channel names\n- Poll data timeout (this has an impact on the\n  data rate indicator\n\nAfter all is initialized, the Data Reader Loop is started"
                    n165 = local read "PRL Configuration"() -> (w381:T1)
                    n166 = Unbundle By Name(w381) -> ("Poll New Data Timeout [ms]"=w380:u16)
                    n167 = call "PRL Access Buffer Writer.vi"("Initialize?"=TRUE) -> ()  [unwired: 7 in, 4 out]
                    n168 = To Long Integer(number=w380) -> (32bit integer=w379:i32)
                    n169 = call "Initialize DLL Readers.vi"("error in (no error)"=w378, "Poll Timeout [5 ms]"=w379, "Phasor Data Concentrator in"=w388) -> ("error out"=w382:errorcluster, "Phasor Data Concentrator out"=w383:refnum<class "Phasor Data Concentrator.lvclass">)  [unwired: 7 in]
                    n170 = call "Initialize Channel Selector.vi"("error in (no error)"=w382, "Phasor Data Concentrator in"=w383) -> ("error out"=w377:errorcluster, "Phasor Data Concentrator out"=w384:refnum<class "Phasor Data Concentrator.lvclass">)  [unwired: 8 in]
                    n171 = Enqueue Element(queue=w387, element="reader;start", error in (no error)=w377) -> (error out=w376:errorcluster)  [unwired: 1 in, 2 out]
                  }
                  frame "start data stream" {
                    n172 = call "PDC Start Data Stream.vi"("error in (no error)"=w390, "Phasor Data Concentrator in"=w392) -> ("error out"=w389:errorcluster, "Phasor Data Concentrator out"=w391:refnum<class "Phasor Data Concentrator.lvclass">)  [unwired: 8 in]
                  }
                  frame "stop data stream" {
                    n173 = call "PDC Stop Data Stream.vi"("error in (no error)"=w394, "Phasor Data Concentrator in"=w396) -> ("error out"=w393:errorcluster, "Phasor Data Concentrator out"=w395:refnum<class "Phasor Data Concentrator.lvclass">)  [unwired: 8 in]
                  }
                  frame "disconnect" {
                    n174 = flat-sequence {
                      tunnel: w402 -> [w407]
                      tunnel: [w406] -> w398
                      tunnel: w400 -> [w404]
                      tunnel: [w403] -> w397
                      tunnel: [w415] -> w401
                      tunnel: w398 -> [w415]
                      tunnel: [w414] -> w399
                      tunnel: w397 -> [w414]
                      frame #0 {
                        # "Don't shutdown the dll if it has\nnot been initialized (this causes\nthe dll to hang for a while)."
                        n175 = local read "PDC Initialized"() -> (w405:bool)
                        n176 = case shown="True" w405 {
                          tunnel: w407 -> [w409 w413]
                          tunnel: [w409 w412] -> w406
                          tunnel: w404 -> [w408 w411]
                          tunnel: [w408 w410] -> w403
                          frame False {
                          }
                          frame True {
                            n177 = call "DLL Disconnect.vi"("error in (no error)"=w411, "Phasor Data Concentrator in"=w413) -> ("error out"=w410:errorcluster, "Phasor Data Concentrator out"=w412:refnum<class "Phasor Data Concentrator.lvclass">)  [unwired: 8 in]
                          }
                        }
                      }
                      frame #1 {
                        w417 = FALSE ("PDC Initialized")
                        n178 = local write "PDC Initialized"(w417) -> ()
                        n179 = local write "PDC Connected"(w417) -> ()
                        n180 = local write "Configuration File Timeout"(w417) -> ()
                        n181 = local write "Configuration File Received"(w417) -> ()
                        n182 = local write "Configuration File Read"(w417) -> ()
                        n183 = local write "Data Rate"(sgl nan ("Data Rate")) -> ()
                      }
                    }
                  }
                }
              }
              frame "reader" {
                n184 = case shown="\"start\"" w422 {
                  tunnel: w421 -> [w426 w432 w438 _ _ _ _]
                  tunnel: w419 -> [w424 w429 w436 w449 w457 w462 w477]
                  tunnel: [w423 w427 w435 w442 w451 w463 w471] -> w418
                  frame "initialize", Default {
                    n185 = Enqueue Element At Opposite End(queue=w426, element="reader;start", error in (no error)=w424) -> (error out=w423:errorcluster)  [unwired: 1 in, 2 out]
                  }
                  frame "start" {
                    n186 = Enqueue Element At Opposite End(queue=w432, element="pdc;start data stream", error in (no error)=w429) -> (queue out=w430:refnum<queue>, error out=w428:errorcluster)  [unwired: 1 in, 1 out]
                    n187 = Enqueue Element(queue=w430, element="reader;set mode logging", error in (no error)=w428) -> (error out=w427:errorcluster)  [unwired: 3 out]
                    "Connected" <- TRUE ("Logging")
                  }
                  frame "stop" {
                    n188 = flat-sequence {
                      frame #0 {
                        n189 = local write "Connected"(FALSE ("Logging")) -> ()
                      }
                      frame #1 {
                        n190 = Wait (ms)(milliseconds to wait=u32 100) -> ()  [unwired: 1 out]
                      }
                    }
                    n191 = Enqueue Element At Opposite End(queue=w438, element="pdc;stop data stream", error in (no error)=w436) -> (error out=w435:errorcluster)  [unwired: 1 in, 2 out]
                  }
                  frame "set mode off" {
                    w441 = T5."Disabled and Grayed Out" ("Disabled")
                    w447 = T5."Enabled" ("Disabled")
                    n192 = property on="Startup" class="Bool"(error in=w449, "DisabledEnum"=w447) -> (error out=w448:errorcluster)  [unwired: 1 in, 1 out]
                    n193 = property on="Config" class="Bool"(error in=w448, "DisabledEnum"=w447) -> (error out=w446:errorcluster)  [unwired: 1 in, 1 out]
                    n194 = property on="Restart" class="Bool"(error in=w446, "DisabledEnum"=w447) -> (error out=w445:errorcluster)  [unwired: 1 in, 1 out]
                    n195 = property on="Shutdown Logging" class="Bool"(error in=w445, "DisabledEnum"=w441) -> (error out=w444:errorcluster)  [unwired: 1 in, 1 out]
                    n196 = property on="Pause" class="Bool (strict)"(error in=w444, "DisabledEnum"=w441) -> (error out=w443:errorcluster)  [unwired: 1 in, 1 out]
                    n197 = property on="Abort Wait" class="Bool (strict)"(error in=w443, "DisabledEnum"=w441) -> (error out=w442:errorcluster)  [unwired: 1 in, 1 out]
                  }
                  frame "set mode startup" {
                    w450 = T5."Disabled and Grayed Out" ("Disabled")
                    n198 = property on="Abort Wait" class="Bool (strict)"(error in=w457, "DisabledEnum"=T5."Enabled" ("Disabled")) -> (error out=w456:errorcluster)  [unwired: 1 in, 1 out]
                    n199 = local write "Abort Wait"(FALSE ("Abort Wait")) -> ()
                    n200 = property on="Config" class="Bool"(error in=w456, "DisabledEnum"=w450) -> (error out=w455:errorcluster)  [unwired: 1 in, 1 out]
                    n201 = property on="Restart" class="Bool"(error in=w455, "DisabledEnum"=w450) -> (error out=w454:errorcluster)  [unwired: 1 in, 1 out]
                    n202 = property on="Shutdown Logging" class="Bool"(error in=w454, "DisabledEnum"=w450) -> (error out=w453:errorcluster)  [unwired: 1 in, 1 out]
                    n203 = property on="Pause" class="Bool (strict)"(error in=w453, "DisabledEnum"=w450) -> (error out=w452:errorcluster)  [unwired: 1 in, 1 out]
                    n204 = property on="Startup" class="Bool"(error in=w452, "DisabledEnum"=w450) -> (error out=w451:errorcluster)  [unwired: 1 in, 1 out]
                  }
                  frame "set mode logging" {
                    w460 = T5."Disabled and Grayed Out" ("Disabled")
                    w461 = T5."Enabled" ("Disabled")
                    n205 = property on="Pause" class="Bool (strict)"(error in=w462, "DisabledEnum"=w461) -> (error out=w468:errorcluster)  [unwired: 1 in, 1 out]
                    n206 = property on="Shutdown Logging" class="Bool"(error in=w468, "DisabledEnum"=w461) -> (error out=w467:errorcluster)  [unwired: 1 in, 1 out]
                    n207 = property on="Config" class="Bool"(error in=w467, "DisabledEnum"=w460) -> (error out=w466:errorcluster)  [unwired: 1 in, 1 out]
                    n208 = property on="Restart" class="Bool"(error in=w466, "DisabledEnum"=w460) -> (error out=w465:errorcluster)  [unwired: 1 in, 1 out]
                    n209 = property on="Abort Wait" class="Bool (strict)"(error in=w465, "DisabledEnum"=w460) -> (error out=w464:errorcluster)  [unwired: 1 in, 1 out]
                    n210 = property on="Startup" class="Bool"(error in=w464, "DisabledEnum"=w460) -> (error out=w463:errorcluster)  [unwired: 1 in, 1 out]
                  }
                  frame "set mode paused" {
                    w469 = T5."Disabled and Grayed Out" ("Disabled")
                    w475 = T5."Enabled" ("Disabled")
                    n211 = property on="Shutdown Logging" class="Bool"(error in=w477, "DisabledEnum"=w475) -> (error out=w476:errorcluster)  [unwired: 1 in, 1 out]
                    n212 = property on="Pause" class="Bool (strict)"(error in=w476, "DisabledEnum"=w475) -> (error out=w473:errorcluster)  [unwired: 1 in, 1 out]
                    n213 = property on="Config" class="Bool"(error in=w473, "DisabledEnum"=w469) -> (error out=w474:errorcluster)  [unwired: 1 in, 1 out]
                    n214 = property on="Restart" class="Bool"(error in=w474, "DisabledEnum"=w469) -> (error out=w470:errorcluster)  [unwired: 1 in, 1 out]
                    n215 = property on="Abort Wait" class="Bool (strict)"(error in=w470, "DisabledEnum"=w469) -> (error out=w472:errorcluster)  [unwired: 1 in, 1 out]
                    n216 = property on="Startup" class="Bool"(error in=w472, "DisabledEnum"=w469) -> (error out=w471:errorcluster)  [unwired: 1 in, 1 out]
                  }
                }
              }
              frame "shutdown" {
                n217 = case shown="\"quit\"" w481 {
                  tunnel: w482 -> [w486 _]
                  tunnel: w479 -> [w484 w490]
                  tunnel: [w483 w489] -> w478
                  frame "", Default {
                    n218 = local write "Shutdown"(TRUE ("Shutdown")) -> ()
                    n219 = call "PRL QUEUE Multiple Elements.vi"("error in"=w484, "Elements to Add"=string[] ["reader;stop", "reader;set mode off", "pdc;disconnect", "shutdown;quit"], "queue"=w486) -> ("error out"=w483:errorcluster)  [unwired: 7 in, 1 out]
                  }
                  frame "quit" {
                    w488 = TRUE ("Quitting...")
                    # "Make sure\nthis loop stops"
                    n220 = Bundle(cluster=w490, "status"=w488) -> (w489:errorcluster)  [unwired: 2 in]
                    "Quitting..." <- w488
                  }
                }
              }
            }
          }
          frame True {
            n221 = local write "Worker Status"(TRUE ("System Ready")) -> ()
            n222 = Wait (ms)(milliseconds to wait=u32 200) -> ()  [unwired: 1 out]
          }
        }
      }
      frame Error {
      }
    }
  }
  n223 = timed-loop {
    timing: w19 -> [_]
    timing-out: [_] -> w18
    shift-right: [w510] -> w15
    shift-left: w16 -> [w511]
    tunnel: w17 -> [w514]
    stop <- w513 stop-if-true
    n224 = node-c288() -> (w505:errorcluster)  [unwired: 1 in]
    n225 = local read "Latest Time Stamp"() -> (w518:timestamp)
    n226 = local read "PRL Configuration"() -> (w507:T1)
    n227 = Unbundle By Name(w507) -> ("Max Time Stamp Age Before Reconnect [s]"=w506:dbl)
    n228 = call "PRL UTIL Check Time Stamp Age.vi"("Max Age Allowed [s]"=5.0, "Time Stamp to Check"=w511) -> ("Trigger"=w517:bool, "Latest Time Stamp"=w512:timestamp)  [unwired: 8 in]
    n229 = call "PRL UTIL Check Time Stamp Age.vi"("Max Age Allowed [s]"=w506, "Time Stamp to Check"=w518) -> ("Trigger"=w516:bool)  [unwired: 8 in, 1 out]
    n230 = local read "Connected"() -> (w508:bool)
    n231 = Compound Arithmetic op=AND(w517, w516, w508) -> (w515:bool)
    n232 = case shown="True" w515 {
      tunnel: w514 -> [_ w524]
      tunnel: w512 -> [_ w523]
      tunnel: w511 -> [w520 _]
      tunnel: [w520 w523] -> w510
      tunnel: w505 -> [w519 w522]
      tunnel: [w519 w521] -> w504
      frame False {
      }
      frame True {
        n233 = disable-structure shown="Enabled" {
          disable-tunnel: w524 -> [w528 _]
          disable-tunnel: w522 -> [w526 w529]
          disable-tunnel: [w525 w529] -> w521
          frame Enabled {
            n234 = call "PRL QUEUE Multiple Elements.vi"("error in"=w526, "Elements to Add"=string[] ["reader;set mode off", "reader;stop", "pdc;disconnect", "pdc;initialize"], "queue"=w528) -> ("error out"=w525:errorcluster)  [unwired: 7 in, 1 out]
          }
          frame Disabled {
            n235 = call <vilib>:"Beep.vi"() -> ()  [unwired: 12 in]
          }
        }
      }
    }
    n236 = local read "Quitting..."() -> (w513:bool)
    n237 = node-c288(w504) -> ()  [unwired: 1 out]
  }
  n238 = flat-sequence {
    tunnel: w24 -> [_]
    tunnel: [w535] -> w20
    tunnel: w17 -> [w535]
    frame #0 {
    }
  }
  n239 = while "Data Reader Loop" {
    tunnel: w20 -> [_]
    tunnel: [w542] -> w26
    shift-right: [w540] -> _
    shift-left: TRUE ("Data?") -> [w541]
    shift-right: [w536] -> w8
    shift-left: w10 -> [_]
    stop <- w542 stop-if-true
    n240 = local read "Connected"() -> (w538:bool)
    n241 = local read "Bad Data Removal"() -> (w539:bool)
    n242 = local read "Queue Active"() -> (w537:bool)
    n243 = case shown="True" w538 {
      tunnel: w541 -> [_ w549]
      tunnel: [TRUE ("Data?") FALSE ("Data?")] -> w540
      tunnel: w539 -> [_ w547]
      tunnel: w537 -> [_ w546]
      frame False {
        n244 = local write "Reader Activity"(0.0 ("Data Rate")) -> ()
        n245 = Wait (ms)(milliseconds to wait=u32 200) -> ()  [unwired: 1 out]
      }
      frame True {
        n246 = stacked-sequence {
          seq-local: [w557 _ _ _] -> [_ w565 _ _]
          seq-local: [w556 _ _ _] -> [_ w563 _ _]
          seq-local: [w555 _ _ _] -> [_ _ w568 _]
          seq-local: [w554 _ _ _] -> [_ _ w570 _]
          seq-local: [w553 _ _ _] -> [_ _ w569 _]
          seq-local: [_ w560 _ _] -> [_ _ _ w573]
          tunnel: w549 -> [w558 _ _ _]
          tunnel: w547 -> [w552 _ _ _]
          tunnel: w546 -> [w551 _ _ _]
          frame #0 {
            n247 = call "PRL Data Reader.vi"("Remove Bad Data?"=w552, "Queue Active?"=w551, "Initialize Time"=w558) -> ("dt (ms)"=w557:dbl, "Buffer Queued?"=w554:bool, "Data Rate"=→"Reader Activity":dbl, "Data?"=w556:bool, "Bad Data?"=w555:bool, "Bad Data Ratio"=w553:dbl, "Latest Time Stamp"=→"Latest Time Stamp":timestamp)  [unwired: 2 in]
            "Data?" <- w556
            "Buffer Queued?" <- w554
          }
          frame #1 {
            n248 = Greater?(x=w565, y="dt max") -> (0:w562:bool)
            n249 = Less?(x=w565, y="dt min") -> (x < y?=w561:bool)
            n250 = Or(x=w562, y=w561) -> (x .or. y?=w564:bool)
            n251 = And(x=w563, y=w564) -> (x .and. y?=w560:bool)
            "Bad dt?" <- w560
          }
          frame #2 {
            n252 = case shown="True" w570 {
              tunnel: w569 -> [_ w572]
              tunnel: w568 -> [_ w571]
              frame False {
              }
              frame True {
                "Complex Bad" <- w572
                "Bad Data?" <- w571
              }
            }
          }
          frame #3 {
            n253 = case shown="True" w573 {
              frame False {
              }
              frame True {
                n254 = local read "Number of bad dt"() -> (w574:u64)
                n255 = Increment(x=w574) -> (x+1=→"Number of bad dt":u64)
              }
            }
          }
        }
      }
    }
    n256 = local read "Quitting..."() -> (w542:bool)
    n257 = call <vilib>:"Clear Errors.vi"() -> ("error out"=w536:errorcluster)  [unwired: 7 in]
  }
  n258 = while "Access Buffer Writer Loop" {
    shift-right: [w578] -> _
    shift-left: FALSE ("Data?") -> [w580]
    tunnel: [w579] -> w21
    tunnel: w20 -> [_]
    shift-right: [w576] -> w7
    shift-left: w10 -> [_]
    stop <- w579 stop-if-true
    n259 = local read "Buffer Active"() -> (w577:bool)
    n260 = Or(x=w577, y=w580) -> (x .or. y?=w578:bool)
    n261 = case shown="False" w578 {
      tunnel: w577 -> [_ w585]
      frame False {
        n262 = Wait (ms)(milliseconds to wait=u32 200) -> ()  [unwired: 1 out]
      }
      frame True {
        n263 = call "PRL Access Buffer Writer.vi"("Write?"=w585) -> ("Lost Data?"=→"Lost File Buffer Data?":bool, "Activity Monitor"=→"Writer Activity":dbl, "Writing?"=→"Writing To File Buffer?":bool)  [unwired: 7 in, 1 out]
      }
    }
    n264 = local read "Quitting..."() -> (w579:bool)
    n265 = call <vilib>:"Clear Errors.vi"() -> ("error out"=w576:errorcluster)  [unwired: 7 in]
  }
  n266 = node-c288(w18) -> ()  [unwired: 1 out]
  n267 = flat-sequence "Shutdown Routine" {
    tunnel: w23 -> [w587]
    tunnel: w15 -> [_]
    tunnel: w6 -> [w586]
    tunnel: [w586] -> w3
    tunnel: [w588] -> w4
    tunnel: w3 -> [w588]
    tunnel: [w589] -> w5
    tunnel: w4 -> [w589]
    tunnel: w20 -> [w593]
    tunnel: [w592] -> w11
    tunnel: w5 -> [w591]
    tunnel: w26 -> [_]
    tunnel: w21 -> [_]
    tunnel: [w594] -> w12
    tunnel: w11 -> [w594]
    frame #0 {
      # "Creates an occation\nin case initialize\nnever got to it."
      n268 = Set Occurrence(w587) -> ()
    }
    frame #1 {
    }
    frame #2 {
      n269 = Wait (ms)(milliseconds to wait=u32 200) -> ()  [unwired: 1 out]
    }
    frame #3 {
      n270 = Release Queue(queue=w593, error in (no error)=w591) -> (error out=w592:errorcluster)  [unwired: 3 out]
    }
    frame #4 {
      w596 = FALSE ("Exit?")
      n271 = local write "Quitting..."(w596) -> ()
      n272 = local write "Shutdown"(w596) -> ()
      n273 = local write "Status"("off" ("Status")) -> ()
    }
  }
  n274 = call <vilib>:"Clear Errors.vi"("error in (no error)"=w2) -> ("error out"=w1:errorcluster)  [unwired: 6 in]
  n275 = Merge Errors(w9, w8, w7, w1) -> (w6:errorcluster)
  "error out" <- w12
